vi "步响应起始点.vi"(3 "eps_rise":dbl=0.001, 4 "step":dbl=10.0, 5 "行程 in":dbl[](array[numeric])) -> (1 "X_value":dbl, 2 "行程 out":dbl[](array[numeric]))   [LabVIEW 2013]
panel:
  in  "（要求）连续大于0的次数":dbl=10.0
  out "连续大于0的次数":dbl=10.0
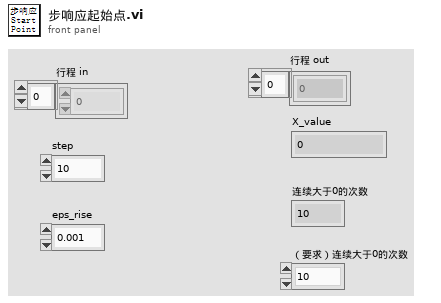
[diagram p1: front panel]
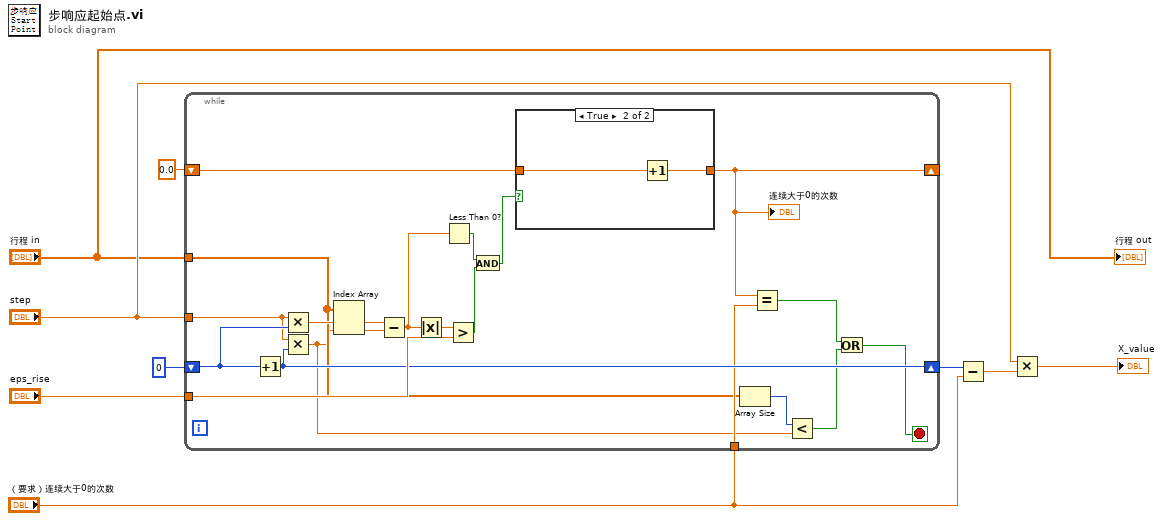
[diagram p0: block diagram]
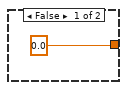
[diagram p2: hidden frame]
diagram:
  n1 = while {
    tunnel: "step" -> [w14]
    tunnel: "行程 in" -> [w19]
    tunnel: "eps_rise" -> [w27]
    shift-right: [w25] -> w3
    shift-left: 0 -> [w26]
    shift-right: [w21] -> _
    shift-left: 0.0 -> [w24]
    tunnel: "（要求）连续大于0的次数" -> [w20]
    stop <- w17 stop-if-true
    n2 = Increment(x=w26) -> (x+1=w25:i32)
    n3 = Multiply(x=w14, y=w26) -> (x*y=w30:dbl)
    n4 = Multiply(x=w14, y=w25) -> (x*y=w13:dbl)
    n5 = Index Array(array=w19, index #1=w30, index #2=w13) -> (element #1=w28:dbl, element #2=w29:dbl)
    n6 = Subtract(x=w28, y=w29) -> (x-y=w12:dbl)
    n7 = Absolute Value(x=w12) -> (abs(x)=w11:dbl)
    n8 = Less Than 0?(x=w12) -> (x < 0?=w23:bool)
    n9 = Greater?(x=w11, y=w27) -> (0:w10:bool)
    n10 = And(x=w23, y=w10) -> (x .and. y?=w22:bool)
    n11 = case shown="True" w22 {
      tunnel: w24 -> [_ w33]
      tunnel: [0.0 w32] -> w21
      frame False {
      }
      frame True {
        n12 = Increment(x=w33) -> (x+1=w32:dbl)
      }
    }
    "连续大于0的次数" <- w21
    n13 = Array Size(array=w19) -> (size(s)=w18:i32)
    n14 = Equal?(x=w21, y=w20) -> (x = y?=w16:bool)
    n15 = Less?(x=w18, y=w13) -> (x < y?=w15:bool)
    n16 = Or(x=w16, y=w15) -> (x .or. y?=w17:bool)
  }
  n17 = Subtract(x=w3, y="（要求）连续大于0的次数") -> (x-y=w1:dbl)
  n18 = Multiply(x="step", y=w1) -> (x*y=→"X_value":dbl)
  "行程 out" <- "行程 in"
